vi "Test Flatten and unflatten Arg.vi"() -> ()   [LabVIEW 2014]
uses:
  user.lib/_NEVSTOP/JKI State Machine ++/JKI-State-Machine-Plus.lvlib
panel:
  out "HEX String (0-9,A-F) 2":string
  out "HEX String (0-9,A-F)":string
  out "Array 2":i32[](array[numeric])=[5, 4, 56, 3, 4]
  in  "Array":i32[](array[numeric])=[577, 33145, 44, 356, 45]
  out "value":T1={"status"=TRUE, "code"=232432, "source"="asdfasdfasdfasvwevweveqv2", "string"="123123qwefqwerf43\n\nasdfasv"}
  in  "error in (no error)":T1={"status"=TRUE, "code"=232432, "source"="asdfasdfasdfasvwevweveqv2", "string"="123123qwefqwerf43\nasdfgb\n\nasdfasv"}
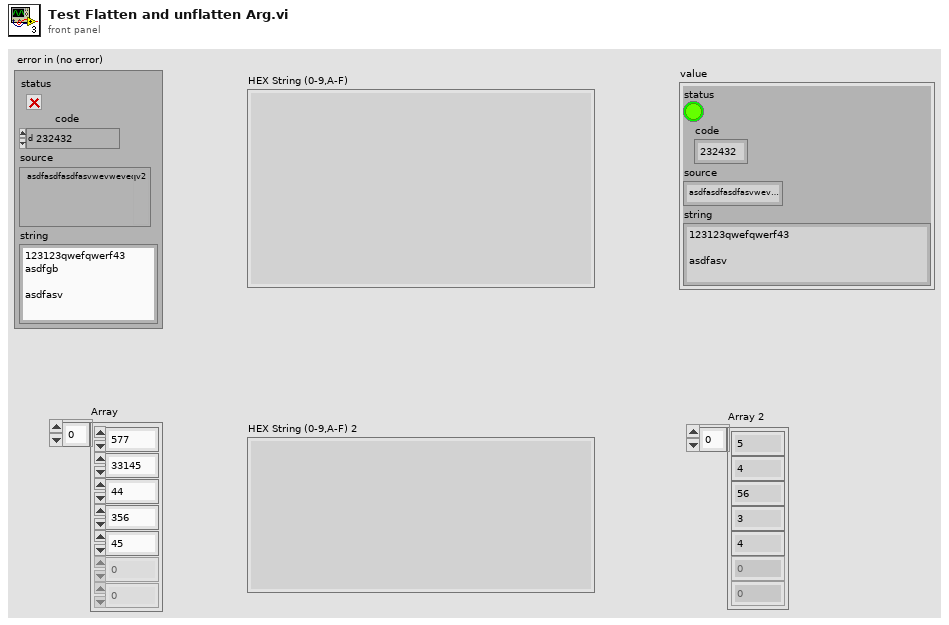
[diagram p1: front panel]
types:
  T1 = cluster{"status":bool, "code":i32, "source":string, "string":string}
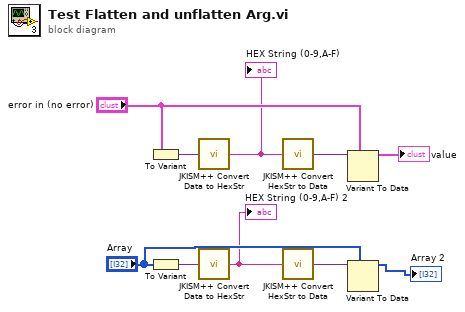
[diagram p0: block diagram]
diagram:
  n1 = To Variant(anything="error in (no error)") -> (Variant=w8:variant)
  n2 = To Variant(anything="Array") -> (Variant=w4:variant)
  n3 = call "JKISM++ Convert Data to HexStr.vi"("Variant"=w8) -> ("HEX String (0-9,A-F)"=w7:string)  [unwired: 8 in]
  "HEX String (0-9,A-F)" <- w7
  n4 = call "JKISM++ Convert Data to HexStr.vi"("Variant"=w4) -> ("HEX String (0-9,A-F)"=w1:string)  [unwired: 8 in]
  "HEX String (0-9,A-F) 2" <- w1
  n5 = call "JKISM++ Convert HexStr to Data.vi"("HEX String"=w7) -> ("Variant"=w6:variant)  [unwired: 8 in]
  n6 = call "JKISM++ Convert HexStr to Data.vi"("HEX String"=w1) -> ("Variant"=w5:variant)  [unwired: 8 in]
  n7 = Variant To Data(type="error in (no error)", Variant=w6) -> (data=→"value":T1)  [unwired: 1 in, 1 out]
  n8 = Variant To Data(type="Array", Variant=w5) -> (data=→"Array 2":i32[])  [unwired: 1 in, 1 out]
